vi "Data To Text.vi"(0 "type descriptor":i16[](array[numeric]) format="%x", 7 "flat data":string, 11 "error in (no error)":errorcluster) -> (8 "text":string, 15 "error out":errorcluster)   [LabVIEW 2012]
uses:
  subvis/private/re_LuaVIEW Push (flat data).vi
  subvis/private/LuaVIEW Pull (string).vi
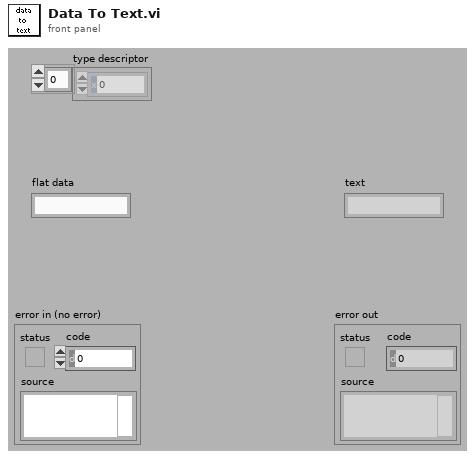
[diagram p1: front panel]
types:
  T1 = typedef "t_LuaVIEW Reference.ctl" = refnum<k1>
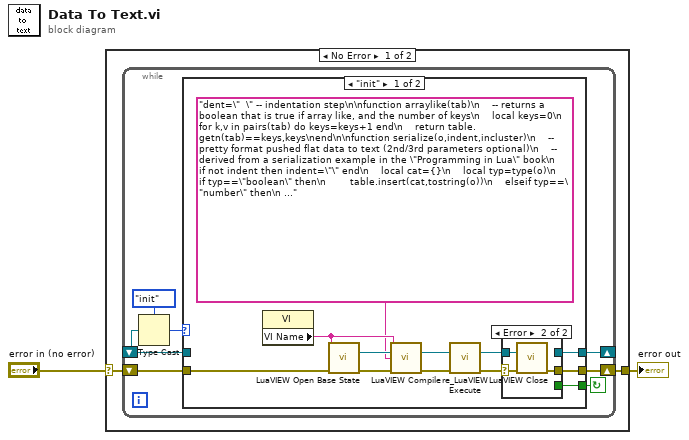
[diagram p0: block diagram]
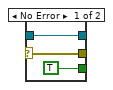
[diagram p2: hidden frame]
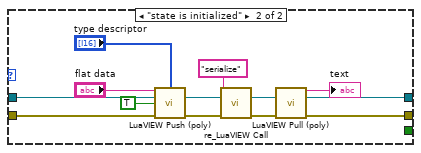
[diagram p3: hidden frame]
diagram:
  n1 = case shown="No Error" "error in (no error)" {
    selector: "error in (no error)" -> [w3 w43]
    tunnel: [w4 w43] -> w2
    frame No Error {
      n2 = while {
        shift-right: [w10] -> _
        shift-left: _ -> [w8]
        shift-right: [w9] -> w4
        shift-left: w3 -> [w11]
        stop <- w5 continue-if-true
        n3 = Type Cast(type=enum32{"init", "state is initialized"}."init", x=w8) -> (*(type *) &x=w6:enum32{"init", "state is initialized"})
        n4 = case shown="\"init\"" w6 {
          tunnel: w11 -> [w23 w42]
          tunnel: [w13 w31] -> w10
          tunnel: [w14 w40] -> w9
          tunnel: w8 -> [_ w41]
          tunnel: [w15 _] -> w5
          frame "init" {
            n5 = property class="VI"() -> ("VI Name"=w19:string)  [unwired: 2 in, 2 out]
            n6 = call "LuaVIEW Open Base State.vi"("close identifier (none)"=w19, "error in (no error)"=w23) -> ("LuaVIEW reference"=w21:T1, "error out"=w17:errorcluster)  [unwired: 12 in]
            n7 = call "LuaVIEW Compile.vi"("script name"=w19, "LuaVIEW reference in"=w21, "script"="dent=\"  \" -- indentation step\n\nfunction arraylike(tab)\n    -- returns a boolean that is true if array like, and the number of keys\n    local keys=0\n    for k,v in pairs(tab) do keys=keys+1 end\n    return table.getn(tab)==keys,keys\nend\n\nfunction serialize(o,indent,incluster)\n    -- pretty format pushed flat data to text (2nd/3rd parameters optional)\n    -- derived from a serialization example in the \"Programming in Lua\" book\n    if not indent then indent=\"\" end\n    local cat={}\n    local typ=type(o)\n    if typ==\"boolean\" then\n        table.insert(cat,tostring(o))\n    elseif typ==\"number\" then\n        if lv.isnan(o) then table.insert(cat,\"_NaN\")\n        elseif lv.isinf(o) then\n            if o>0 then table.insert(cat,\"_Inf\")\n            else table.insert(cat,\"-_Inf\") end\n        else\n            table.insert(cat,tostring(o))\n        end\n    elseif typ==\"string\" then\n        table.insert(cat,string.format(\"%q\",o))\n    elseif typ==\"table\" then\n        local al,keys=arraylike(o)\n        if al and keys == 0 then\n            table.insert(cat,\"{}\")\n        else\n            if incluster then\n                table.insert(cat,\"\\n\"..indent..\"{\\n\")\n            else\n                table.insert(cat,\"{\\n\")\n            end\n            if al then\n                for k,v in ipairs(o) do\n                    table.insert(cat,indent..dent)\n                    table.insert(cat,serialize(v,indent..dent,false))\n                    table.insert(cat,\",\\n\")\n                end\n            else\n                for i,k in ipairs(o._cluster_order) do\n                    table.insert(cat,indent..dent..\"[\"..string.format(\"%q\",k)..\"]=\")\n                    table.insert(cat,serialize(o[k],indent..dent,true))\n                    table.insert(cat,\",\\n\")\n                end\n            end\n            table.insert(cat,indent..\"}\")\n        end\n    else\n        error(\"cannot serialize a \"..type(o))\n    end\n    return table.concat(cat)\nend", "error in (no error)"=w17) -> ("LuaVIEW reference out"=w20:T1, "error out"=w22:errorcluster)  [unwired: 10 in]
            n8 = call "re_LuaVIEW Execute.vi"("LuaVIEW reference in"=w20, "error in (no error)"=w22) -> ("LuaVIEW reference out"=w12:T1, "error out"=w16:errorcluster)  [unwired: 12 in]
            n9 = case shown="Error" w16 {
              selector: w16 -> [w25 w29]
              tunnel: w12 -> [w26 w28]
              tunnel: [w25 w27] -> w14
              tunnel: [w26 _] -> w13
              tunnel: [TRUE _] -> w15
              frame No Error {
              }
              frame Error {
                n10 = call "LuaVIEW Close.vi"("LuaVIEW reference"=w28, "error in (no error)"=w29) -> ("dup error"=w27:errorcluster)  [unwired: 13 in]
              }
            }
          }
          frame "state is initialized" {
            n11 = call-poly "LuaVIEW Push (poly).vi"("flat data"="flat data", "type descriptor"="type descriptor", "LuaVIEW reference in"=w41, "include cluster order (false)"=TRUE, "error in (no error)"=w42) -> ("LuaVIEW reference out"=w38:T1, "error out"=w39:errorcluster)  [unwired: 9 in]
            n12 = call "re_LuaVIEW Call.vi"("function name"="serialize", "LuaVIEW reference in"=w38, "error in (no error)"=w39) -> ("LuaVIEW reference out"=w35:T1, "error out"=w36:errorcluster)  [unwired: 11 in]
            n13 = call-poly "LuaVIEW Pull (poly).vi"("LuaVIEW reference in"=w35, "error in (no error)"=w36) -> ("string"=→"text":string, "LuaVIEW reference out"=w31:T1, "error out"=w40:errorcluster)  [unwired: 11 in]
          }
        }
      }
    }
    frame Error {
    }
  }
  "error out" <- w2
